vi "Manual_Pellet_Dropper.vi"() -> ()   [LabVIEW 2016]
uses:
  <vilib>/LabVIEW Interface for Arduino/Type Defs/Board Type.ctl
  <vilib>/LabVIEW Interface for Arduino/LabVIEW Interface for Arduino.lvlib
panel:
  in  "Hole 6":bool
  in  "Hole 7":bool
  in  "Hole 8":bool
  in  "Hole 9":bool
  in  "Hole 1":bool
  in  "Hole 2":bool
  in  "Hole 3":bool
  in  "Hole 4":bool
  in  "Hole 5":bool
  in  "Drop Pellet":bool
  in  "Terminate":bool
  in  "Stepper Step":i32 min=0 step=1
  in  "# of Pellet":i32=1 max=1000 step=1
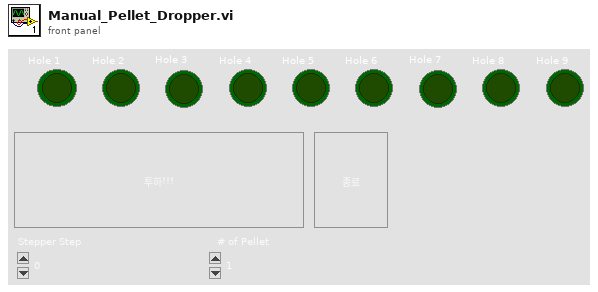
[diagram p1: front panel]
types:
  T1 = typedef "LabVIEW Interface for Arduino.lvlib/Board Type.ctl" = enum16{"Uno", "Dimuelanove w/Atmega 328", "Mega 2560"}
  T2 = typedef "LabVIEW Interface for Arduino.lvlib/Arduino Resource.ctl" = cluster{"VISA resource":refnum<visa-resource-name>, "Board Type":T1, "Connection Type":enum8{"USB / Serial"}, "Bytes Per Packet (15)":u8}
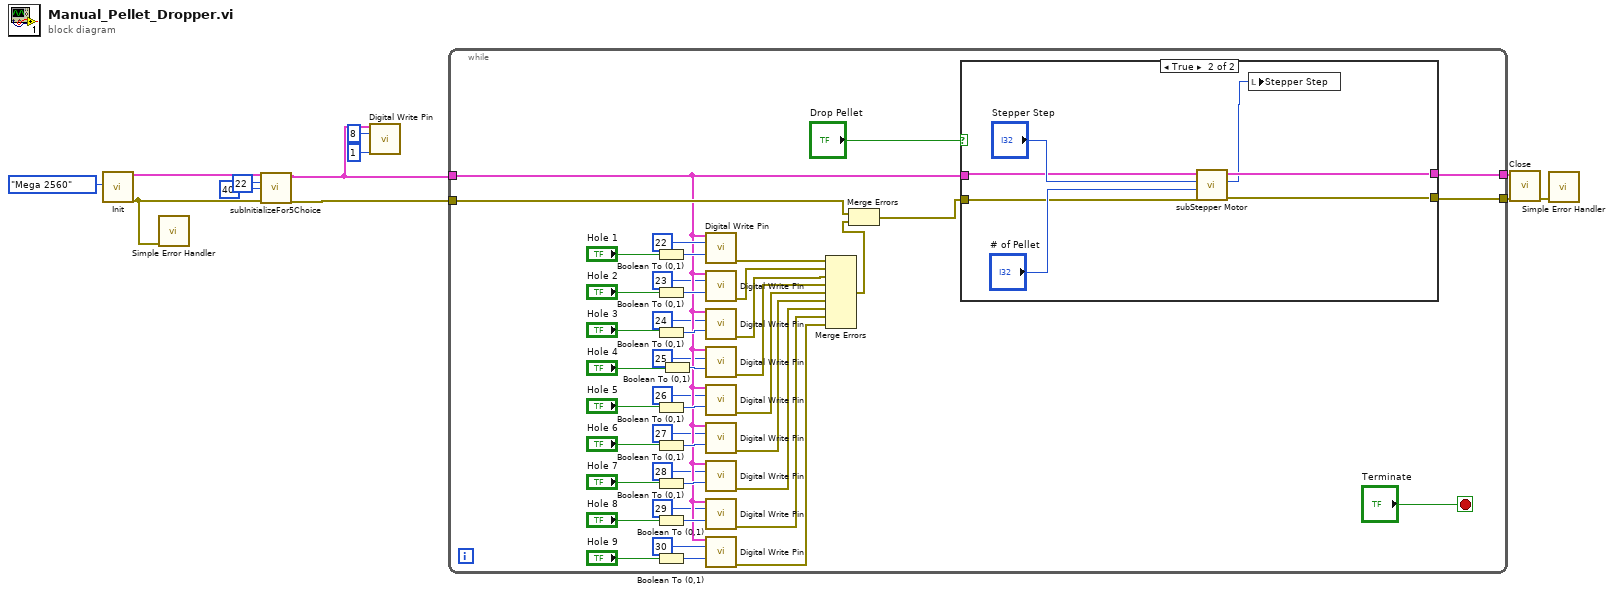
[diagram p0: block diagram]
diagram:
  n1 = call <vilib>:"Init.vi"("Board Type (Uno)"=Board_Type."Mega 2560") -> ("Arduino Resource"=w9:T2, "error out"=w8:errorcluster)  [unwired: 17 in]
  n2 = call <vilib>:"Simple Error Handler.vi"("error in (no error)"=w8) -> ()  [unwired: 4 in, 5 out]
  n3 = call "subInitializeFor5Choice.vi"("Arduino Resource"=w9, "LED Start Pin"=22, "Detector Start Pin"=40, "error in"=w8) -> ("Arduino Resource 2"=w4:T2, "error out"=w5:errorcluster)  [unwired: 10 in]
  n4 = call <vilib>:"Digital Write Pin.vi"("Arduino Resource"=w4, "Digital I/O Pin (0)"=u8 8, "Value (0)"=u8 1) -> ()  [unwired: 11 in, 2 out]
  n5 = while {
    tunnel: w4 -> [w21]
    tunnel: w5 -> [w24]
    tunnel: [w55] -> w12
    tunnel: [w54] -> w11
    stop <- "Terminate" stop-if-true
    n6 = Boolean To (0,1)(Boolean="Hole 1") -> (0, 1=w50:i16)
    n7 = Boolean To (0,1)(Boolean="Hole 2") -> (0, 1=w49:i16)
    n8 = Boolean To (0,1)(Boolean="Hole 3") -> (0, 1=w48:i16)
    n9 = Boolean To (0,1)(Boolean="Hole 5") -> (0, 1=w46:i16)
    n10 = Boolean To (0,1)(Boolean="Hole 6") -> (0, 1=w45:i16)
    n11 = Boolean To (0,1)(Boolean="Hole 7") -> (0, 1=w44:i16)
    n12 = Boolean To (0,1)(Boolean="Hole 8") -> (0, 1=w43:i16)
    n13 = Boolean To (0,1)(Boolean="Hole 9") -> (0, 1=w42:i16)
    n14 = Boolean To (0,1)(Boolean="Hole 4") -> (0, 1=w47:i16)
    n15 = call <vilib>:"Digital Write Pin.vi"("Arduino Resource"=w21, "Digital I/O Pin (0)"=u8 22, "Value (0)"=w50) -> ("error out"=w33:errorcluster)  [unwired: 11 in, 1 out]
    n16 = call <vilib>:"Digital Write Pin.vi"("Arduino Resource"=w21, "Digital I/O Pin (0)"=u8 23, "Value (0)"=w49) -> ("error out"=w32:errorcluster)  [unwired: 11 in, 1 out]
    n17 = call <vilib>:"Digital Write Pin.vi"("Arduino Resource"=w21, "Digital I/O Pin (0)"=u8 24, "Value (0)"=w48) -> ("error out"=w31:errorcluster)  [unwired: 11 in, 1 out]
    n18 = call <vilib>:"Digital Write Pin.vi"("Arduino Resource"=w21, "Digital I/O Pin (0)"=u8 25, "Value (0)"=w47) -> ("error out"=w30:errorcluster)  [unwired: 11 in, 1 out]
    n19 = call <vilib>:"Digital Write Pin.vi"("Arduino Resource"=w21, "Digital I/O Pin (0)"=u8 26, "Value (0)"=w46) -> ("error out"=w29:errorcluster)  [unwired: 11 in, 1 out]
    n20 = call <vilib>:"Digital Write Pin.vi"("Arduino Resource"=w21, "Digital I/O Pin (0)"=u8 27, "Value (0)"=w45) -> ("error out"=w28:errorcluster)  [unwired: 11 in, 1 out]
    n21 = call <vilib>:"Digital Write Pin.vi"("Arduino Resource"=w21, "Digital I/O Pin (0)"=u8 28, "Value (0)"=w44) -> ("error out"=w27:errorcluster)  [unwired: 11 in, 1 out]
    n22 = call <vilib>:"Digital Write Pin.vi"("Arduino Resource"=w21, "Digital I/O Pin (0)"=u8 29, "Value (0)"=w43) -> ("error out"=w26:errorcluster)  [unwired: 11 in, 1 out]
    n23 = call <vilib>:"Digital Write Pin.vi"("Arduino Resource"=w21, "Digital I/O Pin (0)"=u8 30, "Value (0)"=w42) -> ("error out"=w25:errorcluster)  [unwired: 11 in, 1 out]
    n24 = Merge Errors(w33, w32, w31, w30, w29, w28, w27, w26, w25) -> (w23:errorcluster)
    n25 = Merge Errors(w24, w23) -> (w22:errorcluster)
    n26 = case shown="True" "Drop Pellet" {
      tunnel: [w58 w65] -> w55
      tunnel: [w57 w64] -> w54
      tunnel: w21 -> [w58 w60]
      tunnel: w22 -> [w57 w59]
      frame False {
      }
      frame True {
        n27 = call "subStepper Motor.vi"("error in"=w59, "# of Pellet"="# of Pellet", "Numeric"="Stepper Step", "Arduino Resource"=w60) -> ("error out"=w64:errorcluster, "Stepper Step"=w61:i32, "Arduino Resource 2"=w65:T2)  [unwired: 5 in]
        n28 = local write "Stepper Step"(w61) -> ()
      }
    }
  }
  n29 = call <vilib>:"Close.vi"("Arduino Resource"=w12, "error in"=w11) -> ("error out"=w1:errorcluster)  [unwired: 13 in]
  n30 = call <vilib>:"Simple Error Handler.vi"("error in (no error)"=w1) -> ()  [unwired: 4 in, 5 out]
